vi "AtDome_issueCommand_stopShutter.vi"(8 "error in (no error)":errorcluster, 11 "command_stopShutter_Ctl":T1) -> (0 "error out":errorcluster, 2 "function return":i32, 3 "command_stopShutter_Ctl out":T1)   [LabVIEW 2016, in "SALLV_AtDome.lvlib"]
doc: "int AtDome_shm_issueCommand_stopShutterLV(AtDome_command_stopShutterLV *command_stopShutter_Ctl );"
uses:
  SALLV_AtDome.lvlib
  DataTypes/command_stopShutter.ctl
  SALLV_AtDome.so
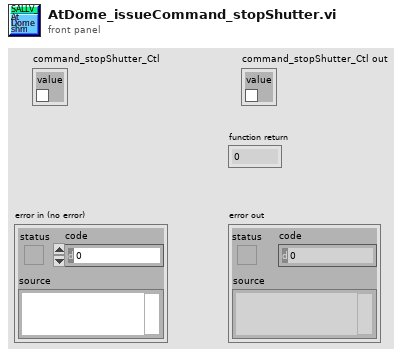
[diagram p1: front panel]
types:
  T1 = typedef "SALLV_AtDome.lvlib/command_stopShutter.ctl" = cluster{"value":bool}
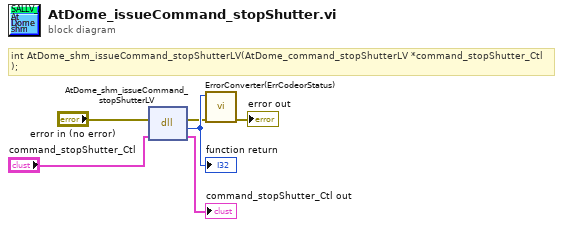
[diagram p0: block diagram]
diagram:
  # "int AtDome_shm_issueCommand_stopShutterLV(AtDome_command_stopShutterLV *command_stopShutter_Ctl );"
  n1 = dll-call lib="home/andres/Desktop/SAL_AtDome/SALLV_AtDome.*" fn="AtDome_shm_issueCommand_stopShutterLV"(error in="error in (no error)", "command_stopShutter_Ctl"="command_stopShutter_Ctl") -> (error out=w2:errorcluster, w6:i32, "command_stopShutter_Ctl"=→"command_stopShutter_Ctl out":T1)  [unwired: 2 in, 1 out]
  "function return" <- w6
  n2 = call "ErrorConverter(ErrCodeorStatus).vi"("error in (no error)"=w2, "error code"=w6) -> ("error out"=→"error out":errorcluster)  [unwired: 9 in]
